vi "DB5000.X读取.vi"(0 "gInitialSIEMENSS7 In":refnum<k24>, 2 "字符识别NG信号":bool=TRUE, 4 "地址数组 2":string[](array[string])=["DB5000.00", "DB5000.100", "DB5000.101", "DB5000.102", "DB5000.103", "DB5000.104", "DB5000.105", "DB5000.106", "DB5000.107", "DB5000.108", "DB5000.109", "DB5000.110", "DB5000.12", "DB5000.13", "DB5000.14", "DB5000.15", "DB5000.16", "DB5000.17", "DB5000.18", "DB5000.19", "DB5000.20", "DB5000.21", "DB5000.22", "DB5000.23", "DB5000.24", "DB5000.25", "DB5000.26", "DB5000.27", "DB5000.28", "DB5000.29", "DB5000.30"], 5 "error in (no error)":errorcluster caption="错误输入（无错误）") -> (3 "组合框":string(combo)="DB5000.01", 14 "gInitialSIEMENSS7 Out":refnum<k24>, 15 "IsSuccess":bool, 16 "结果数组":bool[](array[boolean]), 17 "IO":T2, 19 "error out":errorcluster caption="错误输出")   [LabVIEW 2017]
panel:
  in  "IO 2":T1={"字符识别启动信号-读"=FALSE, "电脑一扫码枪触发-读"=FALSE, "电脑一CCD读取字符触发-读"=FALSE, "电脑一表面检测触发-读"=TRUE, "电脑一穿管检测触发-读"=FALSE, "区间位置1-读"=TRUE, "区间位置2-读"=FALSE, "区间位置3-读"=FALSE, "区间位置4-读"=FALSE, "区间位置5-读"=FALSE, "区间位置6-读"=FALSE, "区间位置7-读"=FALSE, "区间位置8-读"=FALSE, "区间位置9-读"=FALSE, "区间位置10-读"=FALSE, "区间位置11-读"=FALSE, "区间位置12-读"=FALSE, "区间位置13-读"=FALSE, "区间位置14-读"=FALSE, "区间位置15-读"=FALSE, "区间位置16-读"=FALSE, "区间位置17-读"=FALSE, "区间位置18-读"=FALSE, "区间位置19-读"=FALSE, "夹爪1状态-读"=FALSE, "夹爪2状态-读"=FALSE, "夹爪3状态-读"=FALSE, "夹爪4状态-读"=FALSE, "夹爪5状态-读"=FALSE, "夹爪6状态-读"=FALSE, "夹爪7状态-读"=FALSE, "夹爪8状态-读"=FALSE, "夹爪9状态-读"=FALSE, "夹爪10状态-读"=FALSE, "电脑1产品前后位置切换触发-读"=FALSE, "电脑1压力获取触发-读"=FALSE, "PC1 ready-写"=FALSE, "穿管检测pass-写"=FALSE, "表面检测fail-写"=FALSE, "表面检测pass-写"=FALSE, "字符1检测fail-写"=FALSE, "字符1检测pass-写"=FALSE, "混料-写"=FALSE, "数据传递信号-读"=FALSE, "产品尺寸B-写"=FALSE, "产品尺寸A-写"=FALSE, "扫码枪fail-写"=FALSE, "扫码枪pass-写"=FALSE, "穿管检测fail-写"=FALSE, "表面检测完成信号-读"=FALSE, "电脑1衬丝检测触发-读"=FALSE, "表面检测气缸错位-读"=FALSE, "产品尺寸C-写"=FALSE, "PLC初始化-读"=FALSE, "电脑一返工信号-写"=FALSE, "穿管NG停止信号-写"=FALSE, "粗料-写"=FALSE, "细料-写"=FALSE, "短衬丝-写"=FALSE, "长衬丝-写"=FALSE, "衬丝检测fail-写"=FALSE, "衬丝检测pass-写"=FALSE, "一致性检测触发-读"=FALSE}
  out "Content":u8[](array[numeric])
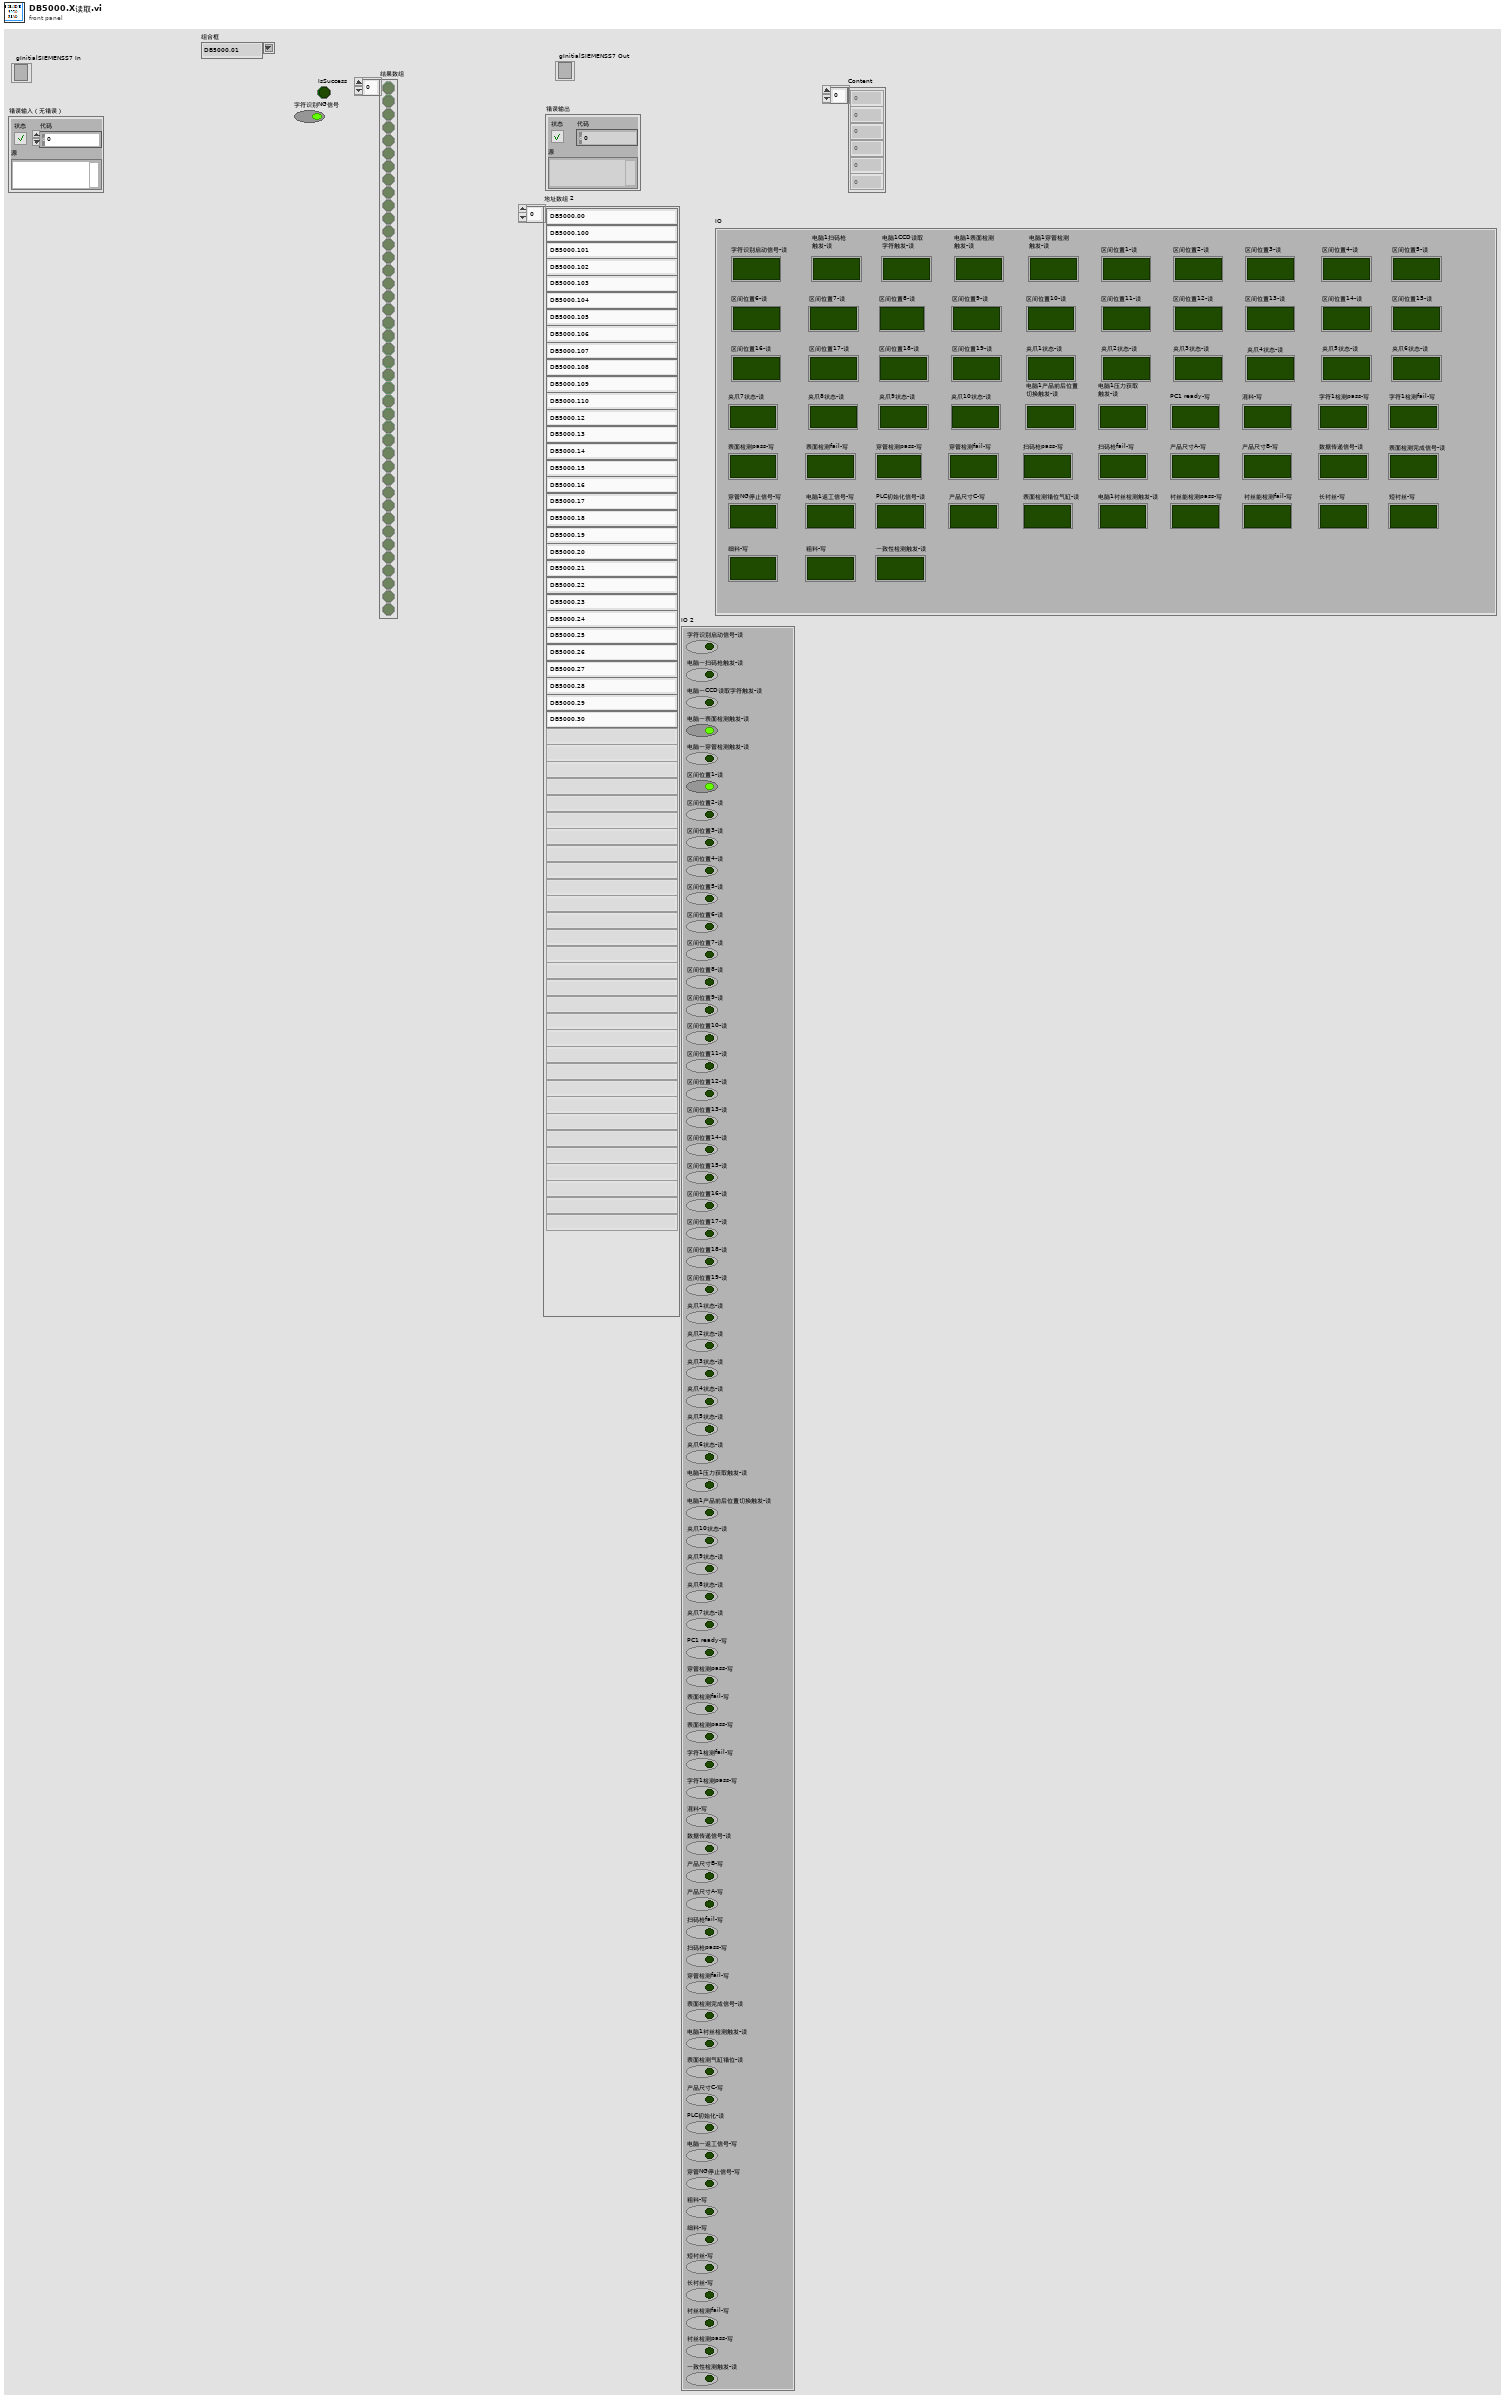
[diagram p1: front panel]
types:
  T1 = cluster{"字符识别启动信号-读":bool, "电脑一扫码枪触发-读":bool, "电脑一CCD读取字符触发-读":bool, "电脑一表面检测触发-读":bool, "电脑一穿管检测触发-读":bool, "区间位置1-读":bool, "区间位置2-读":bool, "区间位置3-读":bool, "区间位置4-读":bool, "区间位置5-读":bool, "区间位置6-读":bool, "区间位置7-读":bool, "区间位置8-读":bool, "区间位置9-读":bool, "区间位置10-读":bool, "区间位置11-读":bool, "区间位置12-读":bool, "区间位置13-读":bool, "区间位置14-读":bool, "区间位置15-读":bool, "区间位置16-读":bool, "区间位置17-读":bool, "区间位置18-读":bool, "区间位置19-读":bool, "夹爪1状态-读":bool, "夹爪2状态-读":bool, "夹爪3状态-读":bool, "夹爪4状态-读":bool, "夹爪5状态-读":bool, "夹爪6状态-读":bool, "夹爪7状态-读":bool, "夹爪8状态-读":bool, "夹爪9状态-读":bool, "夹爪10状态-读":bool, "电脑1产品前后位置切换触发-读":bool, "电脑1压力获取触发-读":bool, "PC1 ready-写":bool, "穿管检测pass-写":bool, "表面检测fail-写":bool, "表面检测pass-写":bool, "字符1检测fail-写":bool, "字符1检测pass-写":bool, "混料-写":bool, "数据传递信号-读":bool, "产品尺寸B-写":bool, "产品尺寸A-写":bool, "扫码枪fail-写":bool, "扫码枪pass-写":bool, "穿管检测fail-写":bool, "表面检测完成信号-读":bool, "电脑1衬丝检测触发-读":bool, "表面检测气缸错位-读":bool, "产品尺寸C-写":bool, "PLC初始化-读":bool, "电脑一返工信号-写":bool, "穿管NG停止信号-写":bool, "粗料-写":bool, "细料-写":bool, "短衬丝-写":bool, "长衬丝-写":bool, "衬丝检测fail-写":bool, "衬丝检测pass-写":bool, "一致性检测触发-读":bool}
  T2 = cluster{"字符识别启动信号-读":bool, "电脑1扫码枪\n触发-读":bool, "电脑1CCD读取\n字符触发-读":bool, "电脑1表面检测\n触发-读":bool, "电脑1穿管检测\n触发-读":bool, "区间位置1-读":bool, "区间位置2-读":bool, "区间位置3-读":bool, "区间位置4-读":bool, "区间位置5-读":bool, "区间位置6-读":bool, "区间位置7-读":bool, "区间位置8-读":bool, "区间位置9-读":bool, "区间位置10-读":bool, "区间位置11-读":bool, "区间位置12-读":bool, "区间位置13-读":bool, "区间位置14-读":bool, "区间位置15-读":bool, "区间位置16-读":bool, "区间位置17-读":bool, "区间位置18-读":bool, "区间位置19-读":bool, "夹爪1状态-读":bool, "夹爪2状态-读":bool, "夹爪3状态-读":bool, "夹爪4状态-读":bool, "夹爪5状态-读":bool, "夹爪6状态-读":bool, "夹爪7状态-读":bool, "夹爪8状态-读":bool, "夹爪9状态-读":bool, "夹爪10状态-读":bool, "电脑1产品前后位置\n切换触发-读":bool, "电脑1压力获取\n触发-读":bool, "PC1 ready-写 ":bool, "混料-写":bool, "字符1检测pass-写":bool, "字符1检测fail-写":bool, "表面检测pass-写":bool, "表面检测fail-写":bool, "穿管检测pass-写":bool, "穿管检测fail-写":bool, "扫码枪pass-写":bool, "扫码枪fail-写":bool, "产品尺寸A-写":bool, "产品尺寸B-写":bool, "数据传递信号-读":bool, "表面检测完成信号-读":bool, "穿管NG停止信号-写":bool, "电脑1返工信号-写":bool, "PLC初始化信号-读":bool, "产品尺寸C-写":bool, "表面检测错位气缸-读":bool, "电脑1衬丝检测触发-读":bool, "衬丝能检测pass-写":bool, "衬丝能检测fail-写":bool, "长衬丝-写":bool, "短衬丝-写":bool, "细料-写":bool, "粗料-写":bool, "一致性检测触发-读":bool}
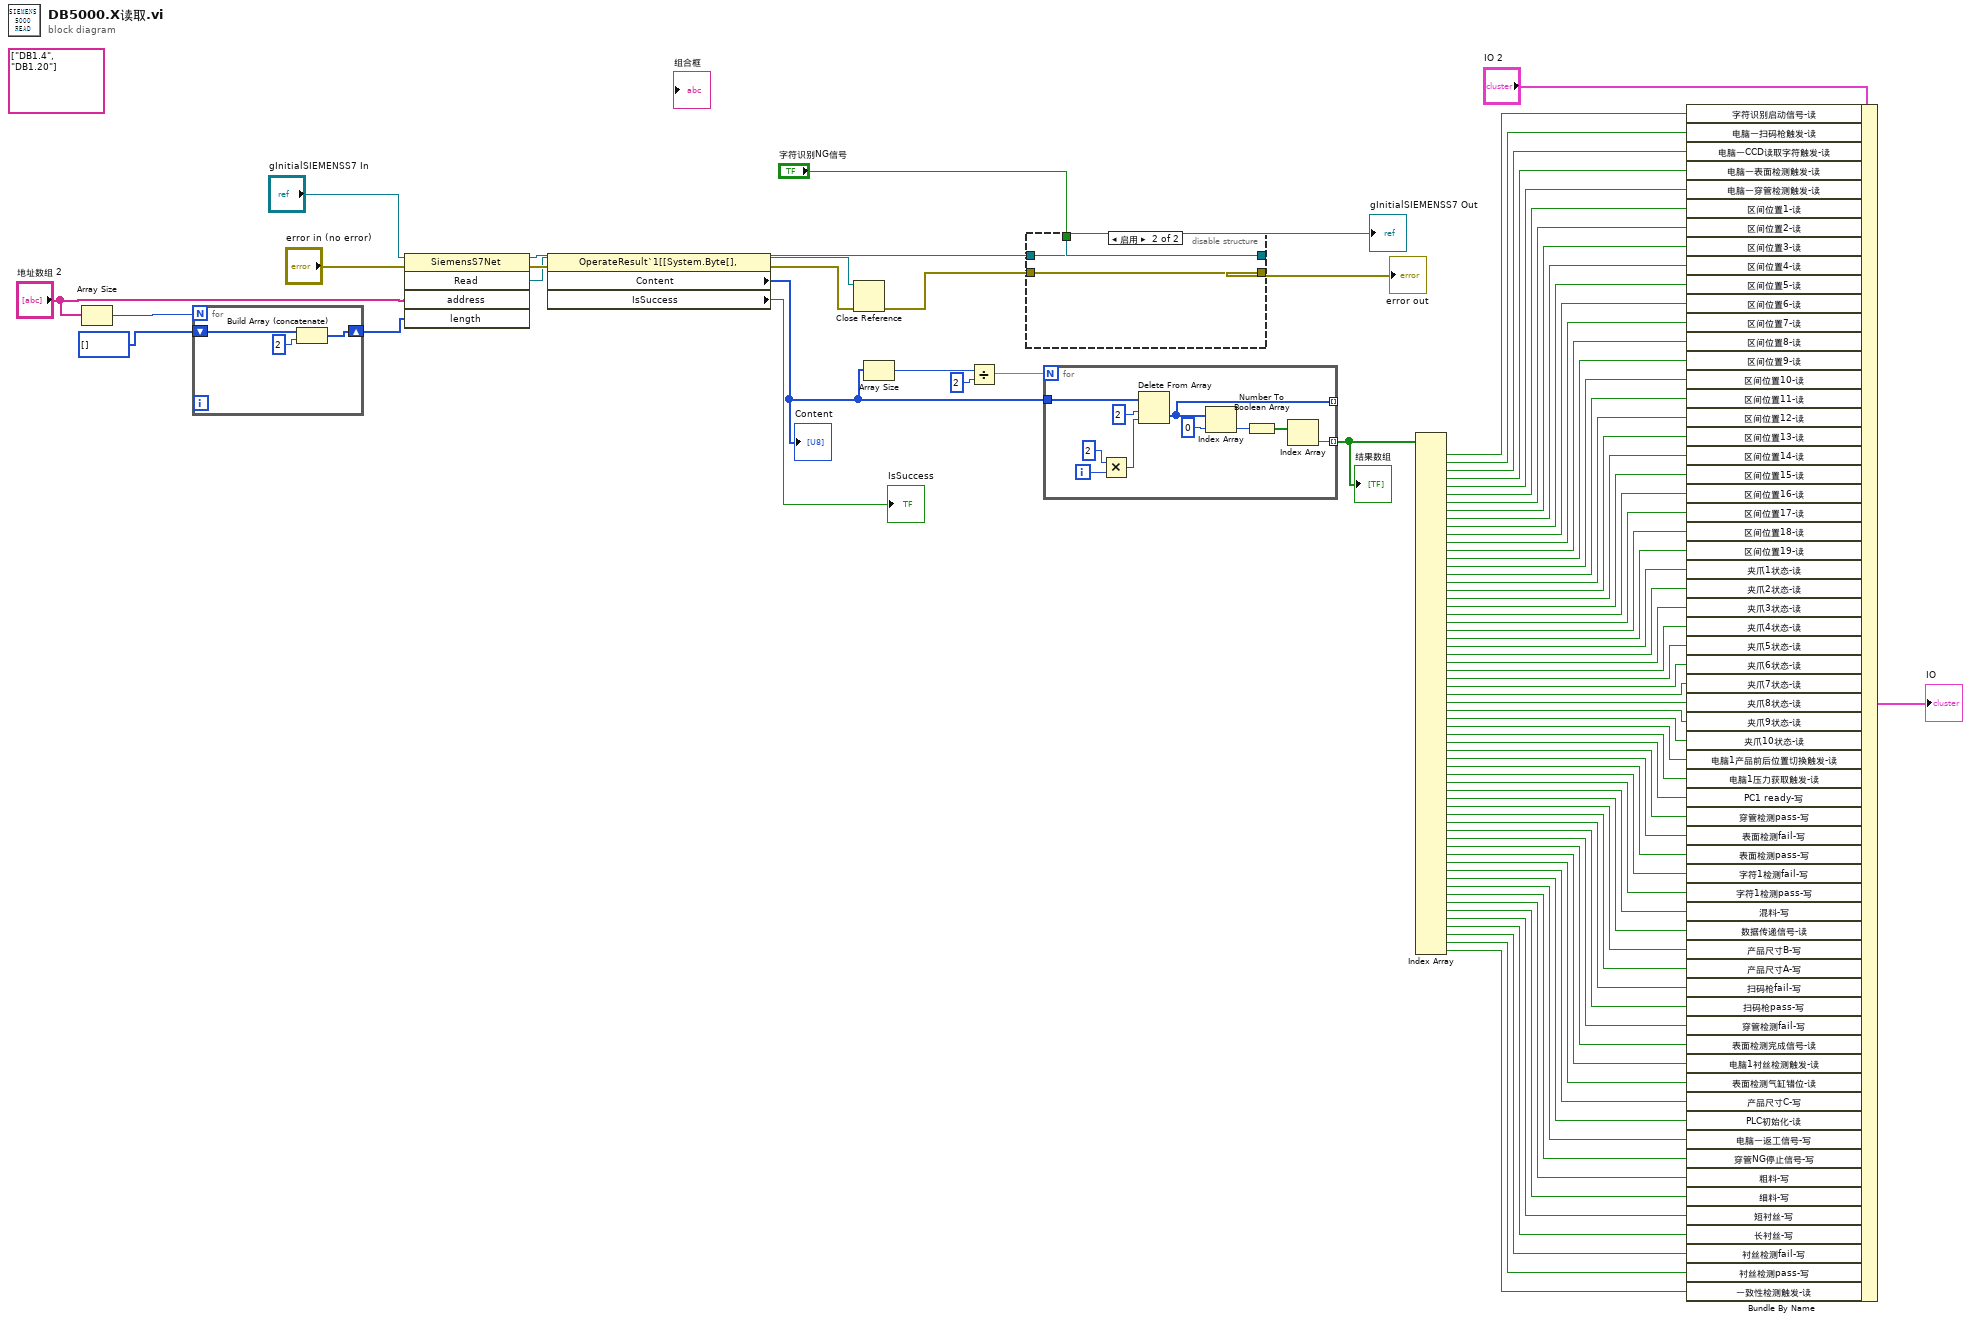
[diagram p0: block diagram]
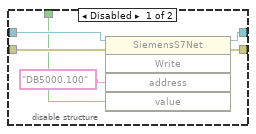
[diagram p2: hidden frame]
diagram:
  (unwired) string[] ["DB1.4", "DB1.20"]
  n1 = Array Size(array="地址数组 2") -> (size(s)=w83:i32)
  n2 = for {
    N: w83 -> [_]
    shift-right: [w88] -> w82
    shift-left: u16[] [] ("添加的数组") -> [w89]
    n3 = Build Array (concatenate)(w89, u16 2) -> (w88:u16[])
  }
  n4 = invoke class="SiemensS7Net" method="Read"(reference="gInitialSIEMENSS7 In", error in="error in (no error)", "address"="地址数组 2", "length"=w82) -> (reference out=w74:refnum<k24>, error out=w85:errorcluster, "Read"=w84:refnum<k24>)  [unwired: 1 in, 2 out]
  n5 = property class="OperateResult`1[[System.Byte[],"(reference=w84, error in=w85) -> (reference out=w3:refnum<k24>, error out=w2:errorcluster, "Content"=w77:u8[], "IsSuccess"=→"IsSuccess":bool)
  "Content" <- w77
  n6 = Close Reference(reference=w3, error in (no error)=w2) -> (error out=w1:errorcluster)
  n7 = Array Size(array=w77) -> (size(s)=w80:i32)
  n8 = Divide(x=w80, y=2) -> (x/y=w78:dbl)
  n9 = disable-structure shown="启用" {
    disable-tunnel: w1 -> [w95 w96]
    disable-tunnel: [w94 w96] -> w75
    disable-tunnel: w74 -> [w93 w97]
    disable-tunnel: [w92 w97] -> w73
    disable-tunnel: "字符识别NG信号" -> [w91 _]
    frame Disabled {
      n10 = invoke class="SiemensS7Net" method="Write"(reference=w93, error in=w95, "address"="DB5000.100" ("组合框"), "value"=w91) -> (reference out=w92:refnum<k24>, error out=w94:errorcluster)  [unwired: 1 in, 3 out]
    }
    frame Enabled {
    }
  }
  "gInitialSIEMENSS7 Out" <- w73
  "error out" <- w75
  n11 = for {
    N: w78 -> [_]
    tunnel: w77 -> [w105]
    tunnel: [w102] -> _ mode=indexing
    tunnel: [w98] -> w76 mode=indexing
    i -> [w107]
    n12 = Multiply(x=2, y=w107) -> (x*y=w103:i32)
    n13 = Delete From Array(array=w105, length=2 ("长度"), index=w103) -> (deleted portion=w102:u8[])  [unwired: 1 out]
    n14 = Index Array(array=w102, index=0 ("索引")) -> (element=w99:u8)
    n15 = Number To Boolean Array(number=w99) -> (Boolean array=w100:bool[])
    n16 = Index Array(array=w100) -> (element=w98:bool)  [unwired: 1 in]
  }
  "结果数组" <- w76
  n17 = Index Array(array=w76) -> (element #1=w71:bool, element #2=w70:bool, element #3=w69:bool, element #4=w68:bool, element #5=w67:bool, element #6=w66:bool, element #7=w65:bool, element #8=w64:bool, element #9=w63:bool, element #10=w62:bool, element #11=w61:bool, element #12=w60:bool, element #13=w59:bool, element #14=w58:bool, element #15=w57:bool, element #16=w56:bool, element #17=w55:bool, element #18=w54:bool, element #19=w53:bool, element #20=w52:bool, element #21=w51:bool, element #22=w50:bool, element #23=w49:bool, element #24=w48:bool, element #25=w47:bool, element #26=w46:bool, element #27=w45:bool, element #28=w44:bool, element #29=w43:bool, element #30=w42:bool, element #31=w41:bool, element #32=w40:bool, element #33=w39:bool, element #34=w38:bool, element #35=w37:bool, element #36=w36:bool, element #37=w35:bool, element #38=w34:bool, element #39=w33:bool, element #40=w32:bool, element #41=w31:bool, element #42=w30:bool, element #43=w29:bool, element #44=w28:bool, element #45=w27:bool, element #46=w26:bool, element #47=w25:bool, element #48=w24:bool, element #49=w23:bool, element #50=w22:bool, element #51=w21:bool, element #52=w20:bool, element #53=w19:bool, element #54=w18:bool, element #55=w17:bool, element #56=w16:bool, element #57=w15:bool, element #58=w14:bool, element #59=w13:bool, element #60=w12:bool, element #61=w11:bool, element #62=w10:bool, element #63=w9:bool)  [unwired: 63 in]
  n18 = Bundle By Name(cluster="IO 2", "字符识别启动信号-读"=w71, "电脑一扫码枪触发-读"=w70, "电脑一CCD读取字符触发-读"=w69, "电脑一表面检测触发-读"=w68, "电脑一穿管检测触发-读"=w67, "区间位置1-读"=w66, "区间位置2-读"=w65, "区间位置3-读"=w64, "区间位置4-读"=w63, "区间位置5-读"=w62, "区间位置6-读"=w61, "区间位置7-读"=w60, "区间位置8-读"=w59, "区间位置9-读"=w58, "区间位置10-读"=w57, "区间位置11-读"=w56, "区间位置12-读"=w55, "区间位置13-读"=w54, "区间位置14-读"=w53, "区间位置15-读"=w52, "区间位置16-读"=w51, "区间位置17-读"=w50, "区间位置18-读"=w49, "区间位置19-读"=w48, "夹爪1状态-读"=w47, "夹爪2状态-读"=w46, "夹爪3状态-读"=w45, "夹爪4状态-读"=w44, "夹爪5状态-读"=w43, "夹爪6状态-读"=w42, "夹爪7状态-读"=w41, "夹爪8状态-读"=w40, "夹爪9状态-读"=w39, "夹爪10状态-读"=w38, "电脑1产品前后位置切换触发-读"=w37, "电脑1压力获取触发-读"=w36, "PC1 ready-写"=w35, "穿管检测pass-写"=w34, "表面检测fail-写"=w33, "表面检测pass-写"=w32, "字符1检测fail-写"=w31, "字符1检测pass-写"=w30, "混料-写"=w29, "数据传递信号-读"=w28, "产品尺寸B-写"=w27, "产品尺寸A-写"=w26, "扫码枪fail-写"=w25, "扫码枪pass-写"=w24, "穿管检测fail-写"=w23, "表面检测完成信号-读"=w22, "电脑1衬丝检测触发-读"=w21, "表面检测气缸错位-读"=w20, "产品尺寸C-写"=w19, "PLC初始化-读"=w18, "电脑一返工信号-写"=w17, "穿管NG停止信号-写"=w16, "粗料-写"=w15, "细料-写"=w14, "短衬丝-写"=w13, "长衬丝-写"=w12, "衬丝检测fail-写"=w11, "衬丝检测pass-写"=w10, "一致性检测触发-读"=w9) -> (→"IO":T1)
